vi "Draw_Sources.vi"(8 "error in (no error)":errorcluster, 11 "IB_SourceTree in":refnum<class "IB_Tree_Source.lvclass">) -> (0 "error out":errorcluster)   [LabVIEW 2020, in "IB_Tree_Source.lvclass"]
uses:
  <vilib>/AppBuilder/IB_Classes/Tree_Source/IB_Tree_Source.lvclass
  <vilib>/AppBuilder/IB_Classes/Tree_Source/IB_Tree_Source.lvclass/IB_Tree_Source.ctl
  <vilib>/AppBuilder/IB_Classes/Tree_Item_Proj_MyComputer/IB_Tree_Item_Proj_MyComputer.lvclass
  <vilib>/AppBuilder/IB_Classes/Tree_Item_Proj_BuildSpecs/IB_Tree_Item_Proj_BuildSpecs.lvclass
  <vilib>/AppBuilder/IB_Classes/Tree/IB_Tree.lvclass
  e:/builds/penguin/labview/branches/2020/dev/dist/vi.lib/AppBuilder/IB_Classes/Tree/IB_Tree.lvclass
  e:/builds/penguin/labview/branches/2020/dev/dist/vi.lib/AppBuilder/IB_Classes/Tree_Source/IB_Tree_Source.lvclass
  e:/builds/penguin/labview/branches/2020/dev/dist/vi.lib/AppBuilder/IB_Classes/Tree_Item_Proj_Container/IB_Tree_Item_Proj_Container.lvclass
  e:/builds/penguin/labview/branches/2020/dev/dist/vi.lib/AppBuilder/IB_Classes/Tree_Item_Proj/IB_Tree_Item_Proj.lvclass
  e:/builds/penguin/labview/branches/2020/dev/dist/vi.lib/AppBuilder/IB_Classes/Tree_Item/IB_Tree_Item.lvclass
  e:/builds/penguin/labview/branches/2020/dev/dist/vi.lib/AppBuilder/IB_Classes/Tree_Item_Proj_MyComputer/IB_Tree_Item_Proj_MyComputer.lvclass
  e:/builds/penguin/labview/branches/2020/dev/dist/vi.lib/AppBuilder/IB_Classes/Tree_Item_Proj_BuildSpecs/IB_Tree_Item_Proj_BuildSpecs.lvclass
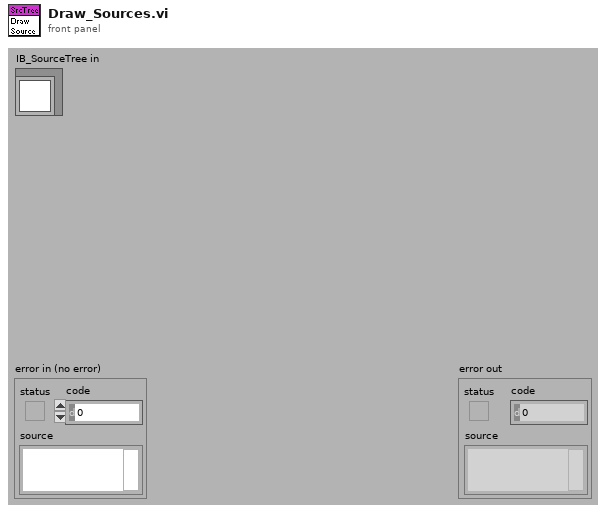
[diagram p1: front panel]
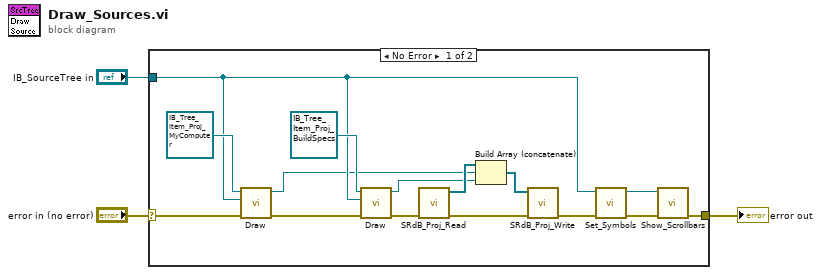
[diagram p0: block diagram]
diagram:
  n1 = case shown="No Error" "error in (no error)" {
    selector: "error in (no error)" -> [w18 w19]
    tunnel: [w11 w19] -> w2
    tunnel: "IB_SourceTree in" -> [w13 _]
    frame No Error {
      n2 = call-dynamic "Draw.vi"("error in (no error)"=w18, "IB_SourceTree in"=w13, "IB_TreeMyComputer in"=refnum<class "IB_Tree_Item_Proj_MyComputer.lvclass"> refnum ("IB_TreeMyComputer.lvclass")) -> ("error out"=w17:errorcluster, "IB_TreeItem out"=w5:refnum<class "IB_Tree_Item_Proj_MyComputer.lvclass">)  [unwired: 7 in]
      n3 = call-dynamic "Draw.vi"("error in (no error)"=w17, "IB_SourceTree in"=w13, "IB_TreeBuildSpecs in"=refnum<class "IB_Tree_Item_Proj_BuildSpecs.lvclass"> refnum ("IB_TreeBuildSpecs.lvclass")) -> ("error out"=w7:errorcluster, "IB_TreeRootItem out"=w4:refnum<class "IB_Tree_Item_Proj_BuildSpecs.lvclass">)  [unwired: 7 in]
      n4 = call <resource>:"SRdB_Proj_Read.vi"("error in (no error)"=w7) -> ("error out"=w8:errorcluster, "Proj Items"=w10:refnum<class "IB_Tree_Item_Proj.lvclass">[])  [unwired: 9 in]
      n5 = Build Array (concatenate)(w10, w5, w4) -> (w9:refnum<class "IB_Tree_Item_Proj.lvclass">[])
      n6 = call <resource>:"SRdB_Proj_Write.vi"("error in (no error)"=w8, "Proj Items"=w9) -> ("error out"=w6:errorcluster)  [unwired: 9 in]
      n7 = call <vilib>:"Set_Symbols.vi"("error in (no error)"=w6, "IB_Tree in"=w13) -> ("error out"=w12:errorcluster, "IB_Tree out"=w14:refnum<class "IB_Tree_Source.lvclass">)  [unwired: 8 in]
      n8 = call <vilib>:"Show_Scrollbars.vi"("error in (no error)"=w12, "IB_Tree in"=w14) -> ("error out"=w11:errorcluster)  [unwired: 8 in, 1 out]
    }
    frame Error {
    }
  }
  "error out" <- w2
